vi "DTReport.vi"   [LabVIEW 2013]
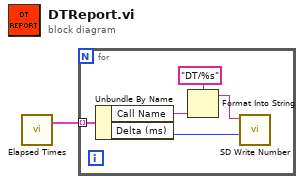
[diagram p0: block diagram]
diagram:
  n1 = call "Elapsed Times.vi"() -> ("Timings"=w1:cluster{"Call Name":string, "Delta (ms)":u32}[])  [unwired: 3 in]
  n2 = for {
    tunnel: w1 -> [w3] mode=indexing
    n3 = Unbundle By Name(w3) -> ("Call Name"=w2:string, "Delta (ms)"=w4:u32)
    n4 = Format Into String(format string="DT/%s" ("Name"), w2) -> (resulting string=w6:string)  [unwired: 2 in, 1 out]
    n5 = call <vilib>:"SD Write Number.vi"("Numeric"=w4, "Name"=w6) -> ()  [unwired: 8 in, 2 out]
  }
